vi "Create Build Specification.vi"(8 "error in (no error)":errorcluster, 10 "Measurement Service Name":string, 11 "Project in":refnum<vi>) -> (0 "error out":errorcluster)   [LabVIEW 2020, in "MeasurementService Editor.lvlib"]
uses:
  MeasurementService Editor.lvlib
  <vilib>/AppBuilder/AB_API/common/AB_API Build Object Selector.ctl
  <vilib>/AppBuilder/AB_API/EXE/NI_AB_API_EXE.lvclass
  <vilib>/AppBuilder/AB_API/common/AB_API Primary Exclusions.ctl
  <vilib>/AppBuilder/AB_API/Build/NI_AB_API_Build.lvclass
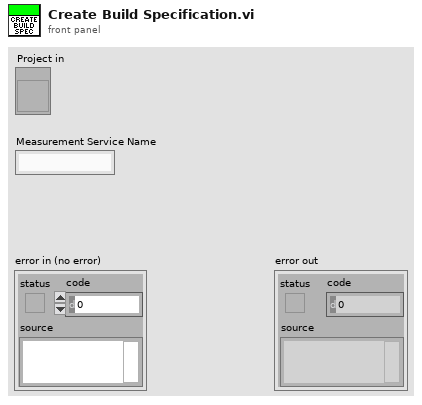
[diagram p1: front panel]
types:
  T1 = typedef "AB_API Build Object Selector.ctl" = enum16{"Source Distribution", "Deployable Source Distribution", "DLL", "EXE", "Packed Library", "Deployable Packed Library", "RT EXE", ".NET Interop Assembly"}
  T2 = typedef "AB_API Primary Exclusions.ctl" = cluster{"Disconnect type definitions":bool, "Remove unused polymorphic VI instances":bool, "Remove unused members of project libraries":bool, "Modify project library file after removing unused members":bool}
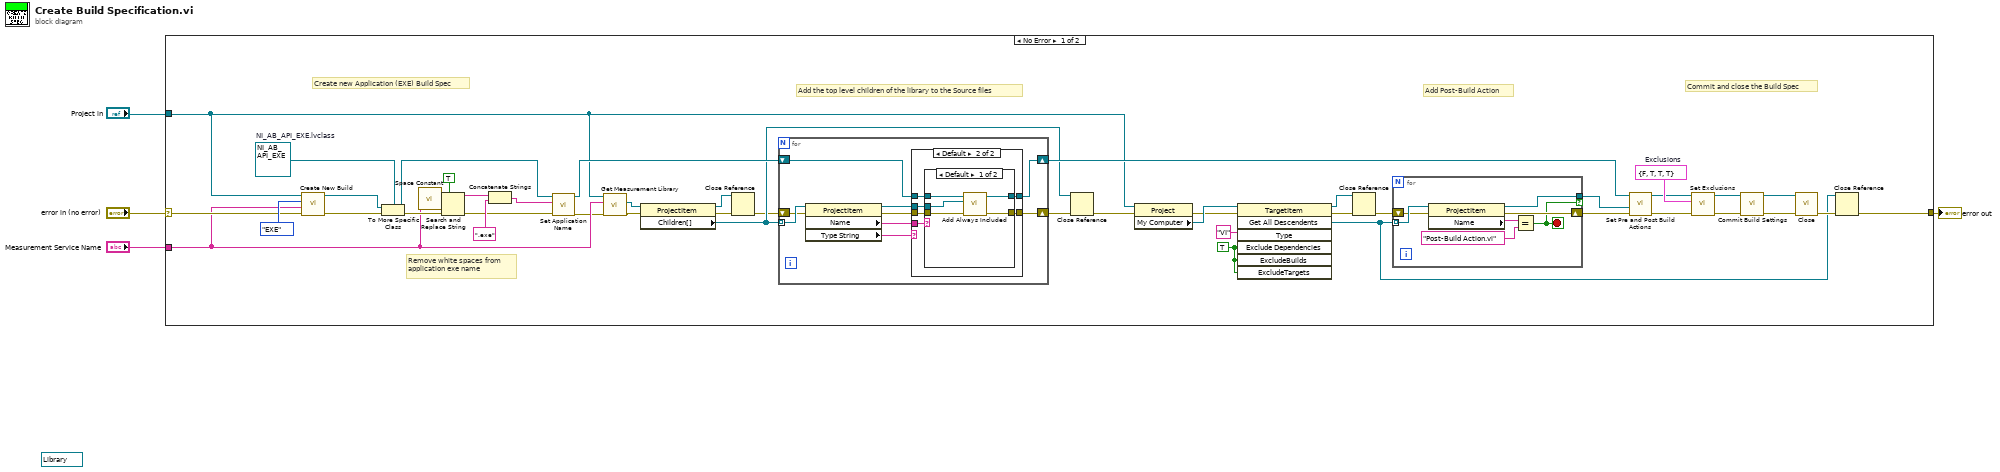
[diagram p0: block diagram]
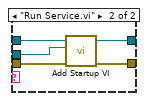
[diagram p3: hidden frame]
diagram:
  (unwired) refnum<vi> refnum ("Library:Open")
  n1 = case shown="No Error" "error in (no error)" {
    selector: "error in (no error)" -> [w48 w84]
    tunnel: "Project in" -> [w13 _]
    tunnel: "Measurement Service Name" -> [w21 _]
    tunnel: [w6 w84] -> w3
    frame No Error {
      w26 = T2 {"Disconnect type definitions"=FALSE, "Remove unused polymorphic VI instances"=TRUE, "Remove unused members of project libraries"=TRUE, "Modify project library file after removing unused members"=TRUE}  # Exclusions
      w30 = TRUE ("ExcludeDependencies")
      w47 = refnum<class "NI_AB_API_EXE.lvclass"> refnum  # NI_AB_API_EXE.lvclass
      # "Remove white spaces from application exe name"
      # "Create new Application (EXE) Build Spec"
      # "Commit and close the Build Spec"
      # "Add Post-Build Action"
      # "Add the top level children of the library to the Source files"
      n2 = call <vilib>:"Create New Build.vi"("error in (no error)"=w48, "Build specification name"=w21, "Build object selector"=AB_API_Build_Object_Selector."EXE", "Project Refnum"=w13) -> ("error out"=w37:errorcluster, "NI_AB_API_Build out"=w46:refnum<class "NI_AB_API_Build.lvclass">)  [unwired: 6 in]
      n3 = To More Specific Class(target class=w47, reference=w46, error in=w37) -> (specific class reference=w40:refnum<class "NI_AB_API_EXE.lvclass">, error out=w36:errorcluster)
      n4 = call <vilib>:"Space Constant.vi"() -> ("String"=w44:string)
      n5 = Search and Replace String(replace all?=TRUE ("replace all? (F)"), input string=w21, search string=w44, error in=w36) -> (result string=w43:string, error out=w35:errorcluster)  [unwired: 4 in, 2 out]
      n6 = Concatenate Strings(w43, ".exe" ("string")) -> (w41:string)
      n7 = call-dynamic "Set Application Name.vi"("error in (no error)"=w35, "Application file name"=w41, "EXE in"=w40) -> ("error out"=w18:errorcluster, "EXE out"=w39:refnum<class "NI_AB_API_EXE.lvclass">)  [unwired: 7 in]
      n8 = call "Get Measurement Library.vi"("error in (no error)"=w18, "Measurement Service Name"=w21, "Project in"=w13) -> ("error out"=w20:errorcluster, "Measurement Library Item"=w19:refnum<vi>)  [unwired: 7 in]
      n9 = property class="ProjectItem"(reference=w19, error in=w20) -> (reference out=w16:refnum<vi>, error out=w15:errorcluster, "Children[]"=w17:refnum<vi>[])
      n10 = Close Reference(reference=w16, error in (no error)=w15) -> (error out=w14:errorcluster)
      n11 = for {
        tunnel: w17 -> [w65] mode=indexing
        shift-right: [w61] -> w38
        shift-left: w39 -> [w63]
        shift-right: [w58] -> w32
        shift-left: w14 -> [w60]
        n12 = property class="ProjectItem"(reference=w65, error in=w60) -> (reference out=w62:refnum<vi>, error out=w59:errorcluster, "Name"=w64:string, "Type String"=w57:string)
        n13 = case shown="Default" w57 {
          tunnel: w64 -> [_ w73]
          tunnel: w63 -> [w67 w72]
          tunnel: w62 -> [_ w71]
          tunnel: [w67 w70] -> w61
          tunnel: w59 -> [w66 w69]
          tunnel: [w66 w68] -> w58
          frame "Folder" {
          }
          frame Default {
            n14 = case shown="Default" w73 {
              tunnel: w72 -> [w78 w83]
              tunnel: w71 -> [w77 w82]
              tunnel: [w76 w81] -> w70
              tunnel: w69 -> [w75 w80]
              tunnel: [w74 w79] -> w68
              frame Default {
                n15 = call-dynamic "Add Always Included.vi"("error in (no error)"=w75, "ProjectItem Refnum"=w77, "EXE in"=w78) -> ("error out"=w74:errorcluster, "EXE out"=w76:refnum<class "NI_AB_API_EXE.lvclass">)  [unwired: 7 in]
              }
              frame "Run Service.vi" {
                n16 = call-dynamic "Add Startup VI.vi"("error in (no error)"=w80, "ProjectItem Refnum"=w82, "EXE in"=w83) -> ("error out"=w79:errorcluster, "EXE out"=w81:refnum<class "NI_AB_API_EXE.lvclass">)  [unwired: 7 in]
              }
            }
          }
        }
      }
      n17 = Close Reference(reference=w17, error in (no error)=w32) -> (error out=w12:errorcluster)
      n18 = property class="Project"(reference=w13, error in=w12) -> (error out=w11:errorcluster, "My Computer"=w27:refnum<vi>)  [unwired: 1 out]
      n19 = invoke class="TargetItem" method="Get All Descendents"(reference=w27, error in=w11, "Type"="VI", "Exclude Dependencies"=w30, "ExcludeBuilds"=w30, "ExcludeTargets"=w30) -> (reference out=w10:refnum<vi>, error out=w9:errorcluster, "All Descendents"=w5:refnum<vi>[])  [unwired: 1 in, 4 out]
      n20 = Close Reference(reference=w10, error in (no error)=w9) -> (error out=w8:errorcluster)
      n21 = for {
        tunnel: w5 -> [w56] mode=indexing
        shift-right: [w53] -> w28
        shift-left: w8 -> [w51]
        tunnel: [w52] -> w29 if=w50
        stop <- w50 stop-if-true
        n22 = property class="ProjectItem"(reference=w56, error in=w51) -> (reference out=w52:refnum<vi>, error out=w53:errorcluster, "Name"=w54:string)
        n23 = Equal?(x=w54, y="Post-Build Action.vi") -> (x = y?=w50:bool)
      }
      n24 = call-dynamic "Set Pre and Post Build Actions.vi"("error in (no error)"=w28, "Post Build Action VI"=w29, "Build in"=w38) -> ("error out"=w23:errorcluster, "Build out"=w25:refnum<class "NI_AB_API_EXE.lvclass">)  [unwired: 7 in]
      n25 = call-dynamic "Set Exclusions.vi"("error in (no error)"=w23, "Exclusions"=w26, "EXE in"=w25) -> ("error out"=w22:errorcluster, "EXE out"=w24:refnum<class "NI_AB_API_EXE.lvclass">)  [unwired: 7 in]
      n26 = call-dynamic "Commit Build Settings.vi"("error in (no error)"=w22, "EXE in"=w24) -> ("error out"=w33:errorcluster, "EXE out"=w34:refnum<class "NI_AB_API_EXE.lvclass">)  [unwired: 8 in]
      n27 = call-dynamic "Close.vi"("error in (no error)"=w33, "EXE in"=w34) -> ("error out"=w7:errorcluster)  [unwired: 9 in]
      n28 = Close Reference(reference=w5, error in (no error)=w7) -> (error out=w6:errorcluster)
    }
    frame Error {
    }
  }
  "error out" <- w3
